vi "workbook.scope_rid_at.vi"(8 "error in":errorcluster, 11 "Workbook in":refnum<class "Workbook.lvclass">) -> (0 "error out":errorcluster, 3 "Workbook out":refnum<class "Workbook.lvclass">)   [LabVIEW 2020, in "Workbook.lvclass"]
doc: "Returns the asset or run RID at the given position in the workbook's data scope."
uses:
  Workbook.lvclass
  Workbook.lvclass/Workbook.ctl
  client.lvlib
panel:
  out "out_needed out":u32
  out "scope rid":string
  in  "index":i32
  in  "buf":string
  in  "cap":u32
  in  "out_needed":u32
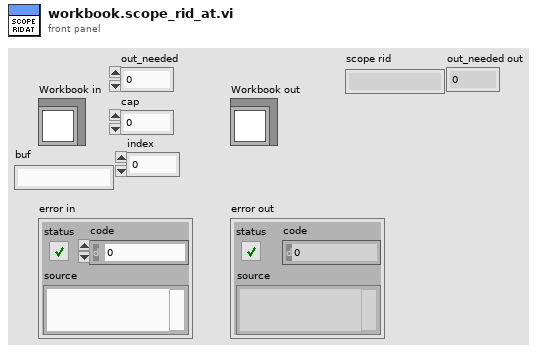
[diagram p1: front panel]
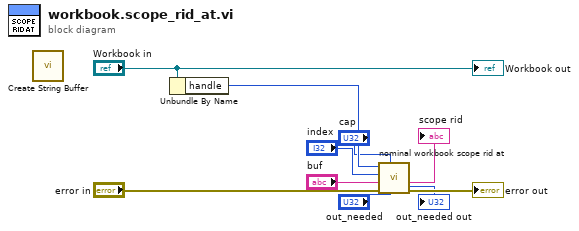
[diagram p0: block diagram]
diagram:
  n1 = call "Create String Buffer.vi"() -> ()  [unwired: 9 in, 3 out]
  n2 = Unbundle By Name("Workbook in") -> ("handle"=w8:i32)
  n3 = call "nominal workbook scope rid at.vi"("out_needed"="out_needed", "cap"="cap", "error in (no error)"="error in", "buf"="buf", "index"="index", "workbook"=w8) -> ("error out"=→"error out":errorcluster, "buf out"=→"scope rid":string, "out_needed out"=→"out_needed out":u32)  [unwired: 2 in, 1 out]
  "Workbook out" <- "Workbook in"
